vi "Add bulk rows.vi"(8 "error in (no error)":errorcluster, 10 "Item Names":string[][](array[string]), 11 "MulColLBTable.lvclass":refnum<class "MulColLBTable.lvclass">) -> (0 "error out":errorcluster, 3 "MulColLBTable.lvclass 2":refnum<class "MulColLBTable.lvclass">)   [LabVIEW 2020, in "MulColLBTable.lvclass"]
uses:
  MulColLBTable.lvclass
  MulColLBTable.lvclass/MulColLBTable.ctl
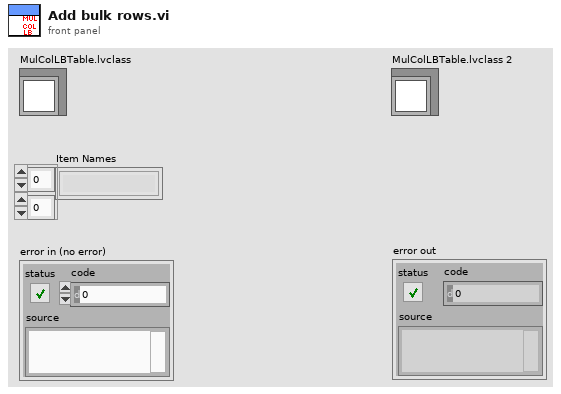
[diagram p1: front panel]
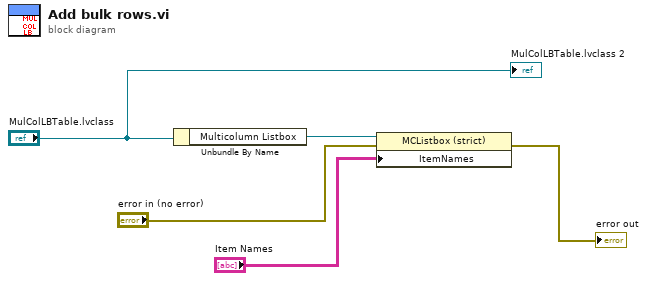
[diagram p0: block diagram]
diagram:
  n1 = Unbundle By Name("MulColLBTable.lvclass") -> ("Multicolumn Listbox"=w4:refnum<vi>)
  n2 = property class="MCListbox (strict)"(reference=w4, error in="error in (no error)", "ItemNames"="Item Names") -> (error out=→"error out":errorcluster)  [unwired: 1 out]
  "MulColLBTable.lvclass 2" <- "MulColLBTable.lvclass"
